vi "Proportional.vi"(8 "error in (no error)":errorcluster, 11 "PID in":refnum<class "PID.lvclass">) -> (0 "error out":errorcluster, 3 "PID out":refnum<class "PID.lvclass">)   [LabVIEW 2024, in "PID.lvlib" / "PID.lvclass"]
uses:
  PID.lvclass
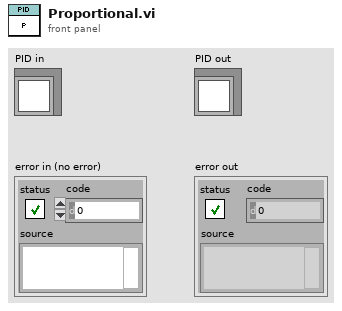
[diagram p1: front panel]
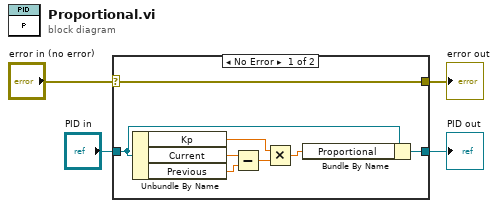
[diagram p0: block diagram]
diagram:
  n1 = case shown="No Error" "error in (no error)" {
    selector: "error in (no error)" -> [w12 w14]
    tunnel: [w12 w14] -> w3
    tunnel: [w5 w13] -> w1
    tunnel: "PID in" -> [w7 w13]
    frame No Error {
      n2 = Unbundle By Name(w7) -> ("Kp"=w9:dbl, "Current"=w11:dbl, "Previous"=w10:dbl)
      n3 = Subtract(x=w11, y=w10) -> (x-y=w8:dbl)
      n4 = Multiply(x=w9, y=w8) -> (x*y=w6:dbl)
      n5 = Bundle By Name(cluster=w7, "Proportional"=w6) -> (w5:refnum<class "PID.lvclass">)
    }
    frame Error {
    }
  }
  "error out" <- w3
  "PID out" <- w1
